vi "tester1.vi"() -> ()   [LabVIEW 2009]
panel:
  out "Column Headers":T1
  out "2D Data Array":string[][](array[string])
  in  "Run Name":string
  in  "Valve Name":string
  in  "Board Name":string
  in  "Waveform Array Input":T2(array[cluster])
  out "Waveform Array":T3(array[cluster])
  in  "Build Interval (ms)":dbl
  in  "Waveform Input":waveform(dbl)
  in  "Max Elapsed Build Time (ms)":dbl
  out "concatenated string":string
  in  "Clear Trigger SP Latch":bool=TRUE
  out "PASS/FAIL Value":bool
  in  "Clear PASS/FAIL Selection":bool
  out "FAIL Pulse":bool
  out "PASS Pulse":bool
  out "PASS OR FAIL Pulse":bool
  in  "FAIL Button":bool
  in  "PASS Button":bool
  out "Waveform Output":waveform(dbl)
  in  "High Trigger SP (VDC)":dbl
  out "Elapsed ms":dbl
  in  "y":i32
  out "Loops/Second":dbl
  out "Loop Count":i32
  out "Y":dbl[](array[numeric])
  out "Waveform Chart 2":waveform(dbl)(graph)
  in  "E-STOP Input":bool
  in  "Module Configure":T4={"DAQ #"=1, "Module #"=4, "Samples"=1000, "Mode"=10178, "Rate (Hz)"=1000.0, "Min VDC"=-10.0, "Max VDC"=32.0, "Module Type"=enum."CDAQ"} {"Rate (Hz)" format="%0.2f"; "Mode" items=["Finite Samples"=10178, "Continuous Samples"=10123, "Hardware Timed Single Point"=12522]}
  out "Task OUT":refnum<k21>="cDAQ1Mod4"
  out "Error OUT":errorcluster
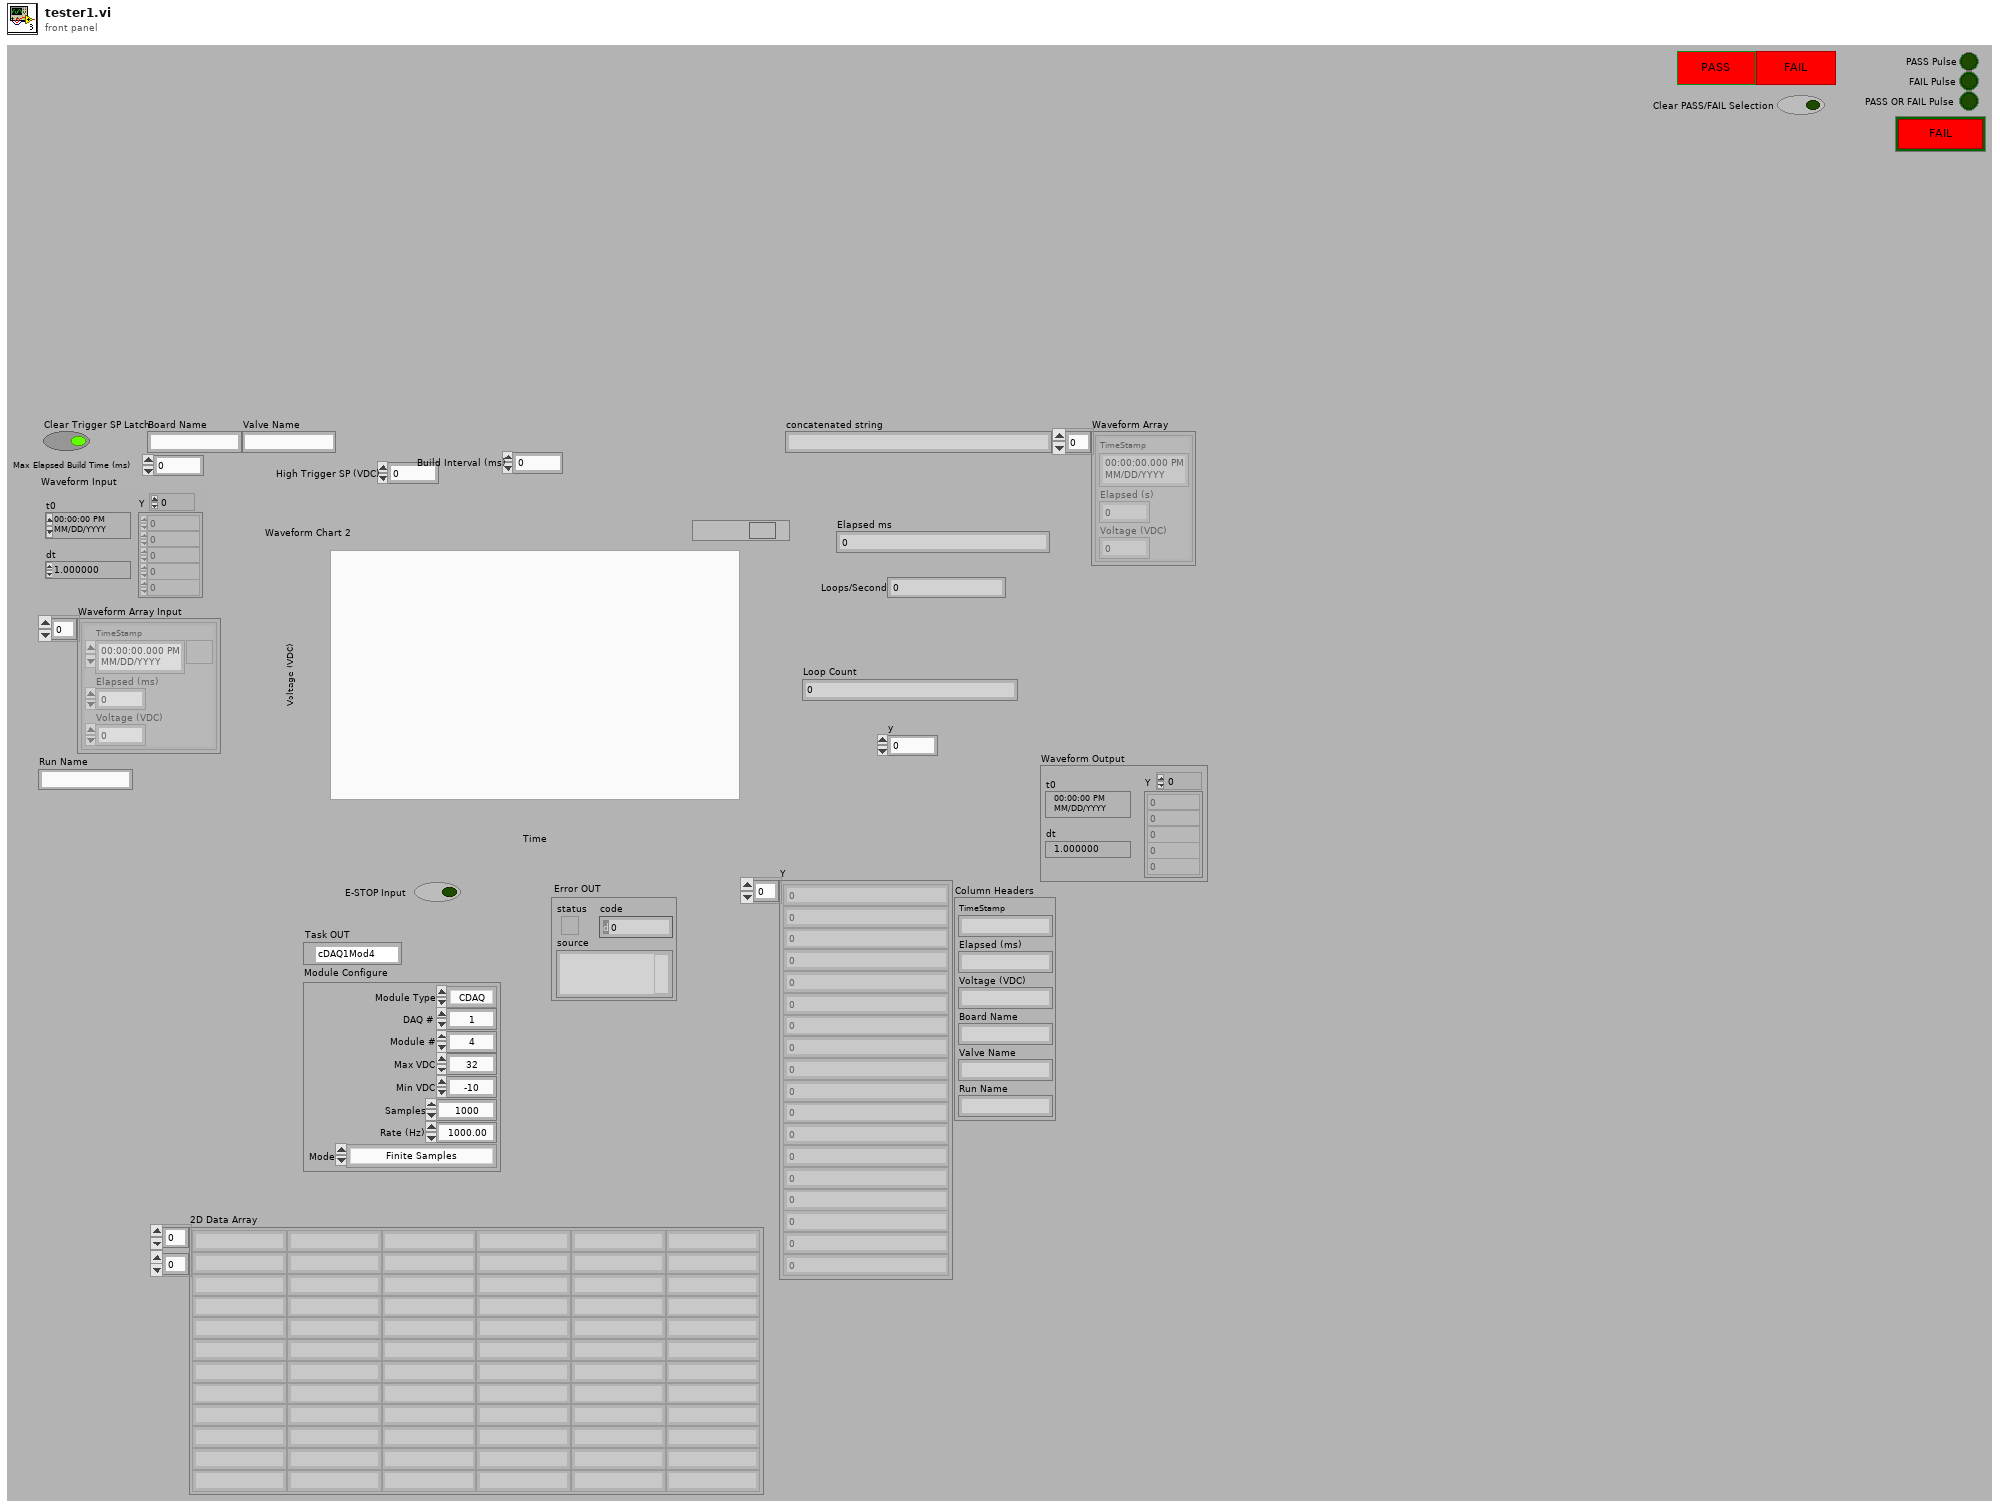
[diagram p1: front panel]
types:
  T1 = cluster{"TimeStamp":string, "Elapsed (ms)":string, "Voltage (VDC)":string, "Board Name":string, "Valve Name":string, "Run Name":string}
  T2 = cluster{"TimeStamp":timestamp, "Elapsed (ms)":dbl, "Voltage (VDC)":dbl}[]
  T3 = cluster{"TimeStamp":timestamp, "Elapsed (s)":dbl, "Voltage (VDC)":dbl}[]
  T4 = cluster{"DAQ #":i32, "Module #":i32, "Samples":i32, "Mode":i32, "Rate (Hz)":dbl, "Min VDC":dbl, "Max VDC":dbl, "Module Type":enum16{"CDAQ", "SCXI"}}
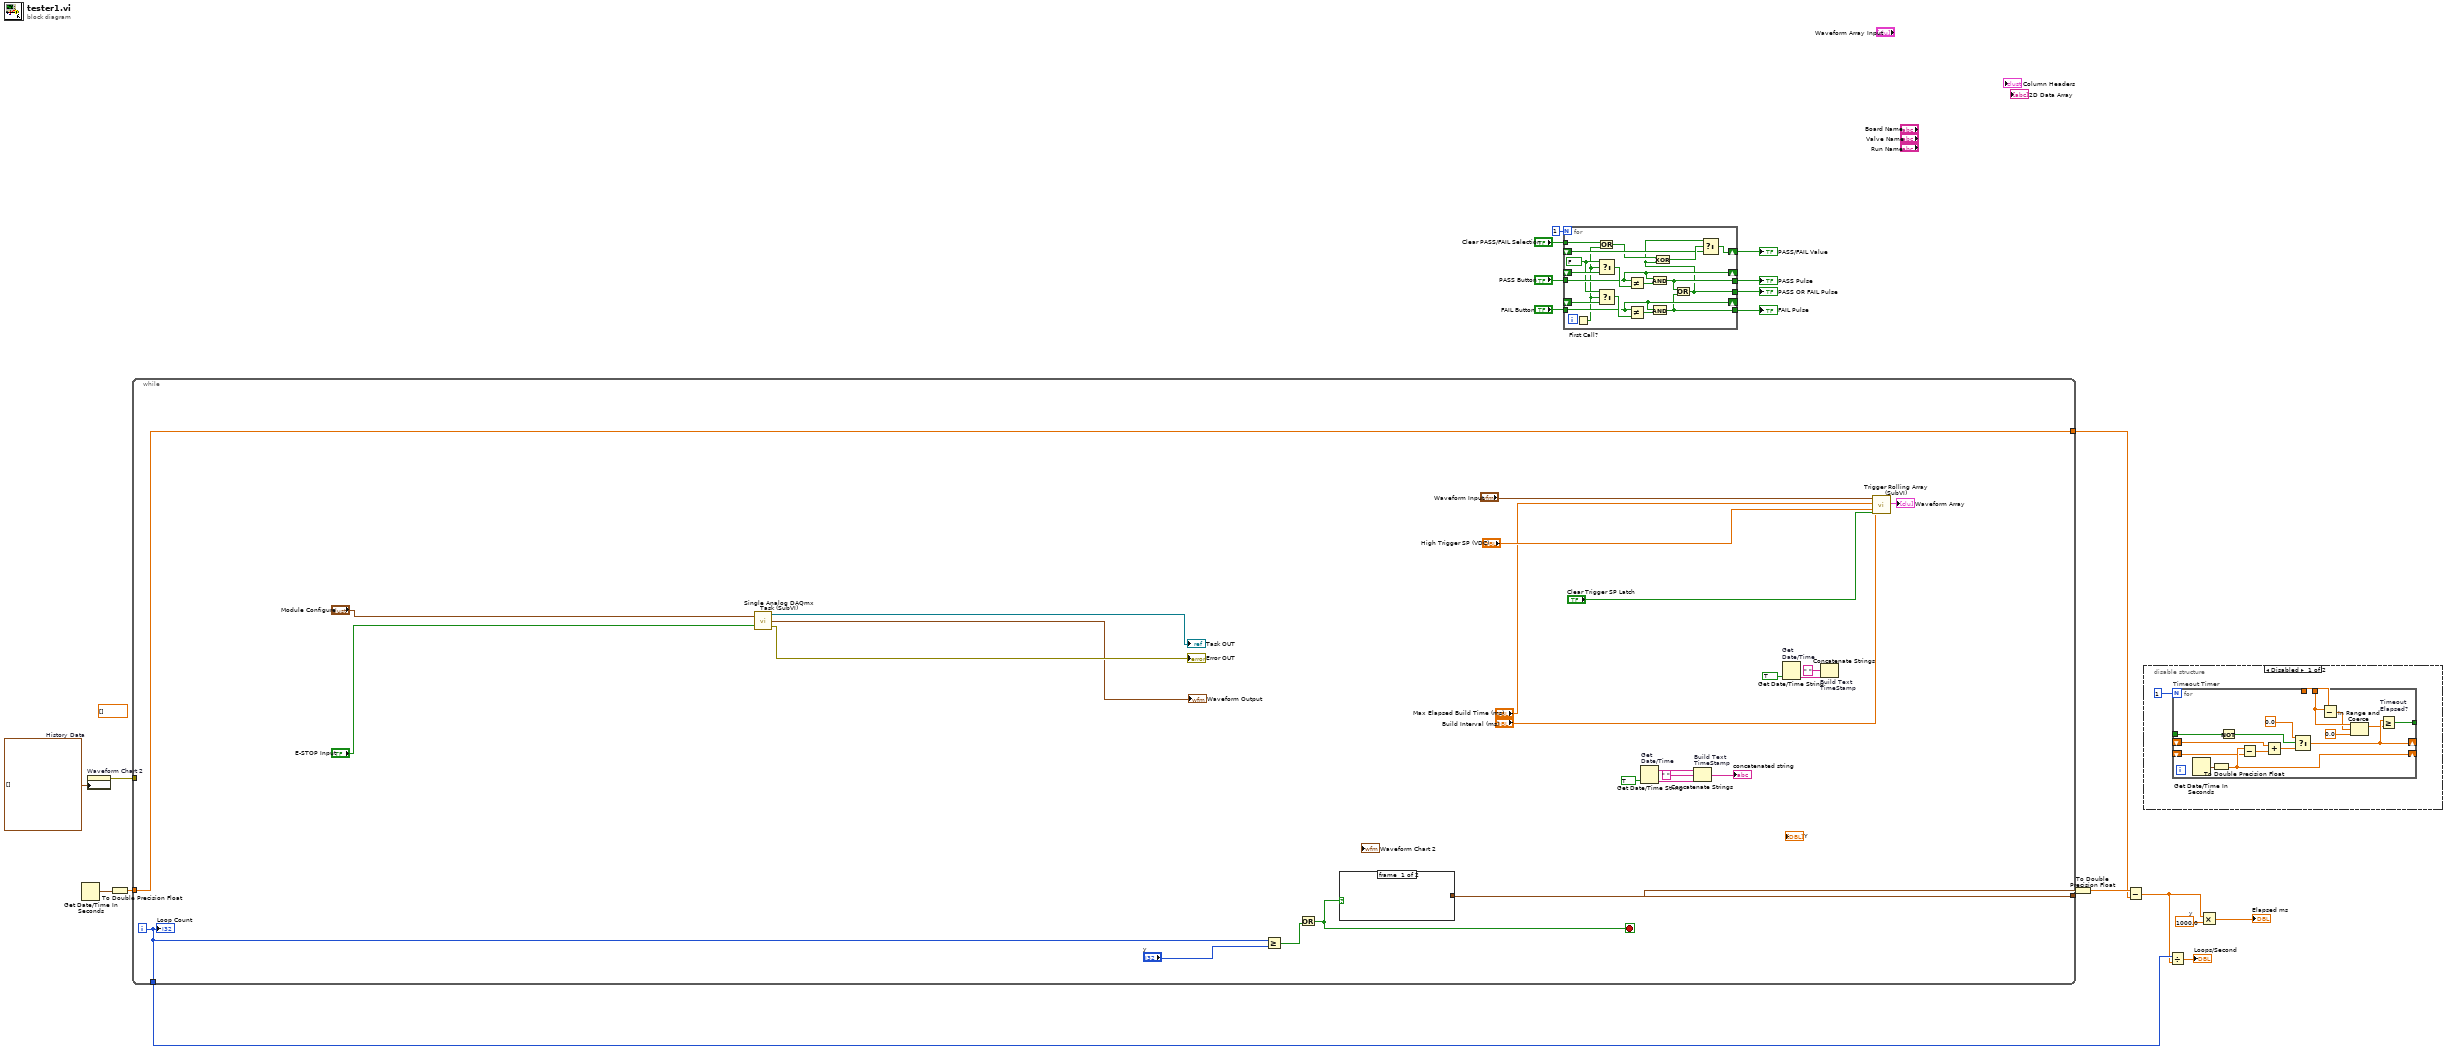
[diagram p0: block diagram]
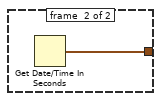
[diagram p3: hidden frame]
diagram:
  w10 = 1000.0  # y
  w19 = waveform(dbl)[] []  # History Data
  (unwired) dbl[] []
  n1 = Get Date/Time In Seconds() -> (seconds since 1Jan1904=w18:timestamp)
  n2 = property on="Waveform Chart 2" class="WFChart (strict)"("History Data"=w19) -> (error out=w20:errorcluster)  [unwired: 2 in, 1 out]
  n3 = To Double Precision Float(number=w18) -> (double precision float=w17:dbl)
  n4 = while {
    tunnel: w20 -> [_]
    tunnel: w17 -> [w44]
    tunnel: [w44] -> w14
    tunnel: [w43] -> w16
    tunnel: [w39] -> w12
    i -> [w39]
    stop <- w38 stop-if-true
    n5 = call "Single Analog DAQmx Task (SubVI).vi"("Module Configure"="Module Configure", "E-STOP Input"="E-STOP Input") -> ("Task OUT"=→"Task OUT":refnum<k21>, "Waveform Output"=→"Waveform Output":waveform(dbl), "Error OUT"=→"Error OUT":errorcluster)
    n6 = Greater Or Equal?(x=w39, y="y") -> (x >= y?=w41:bool)
    n7 = Or(y=w41) -> (x .or. y?=w38:bool)  [unwired: 1 in]
    n8 = case shown="True" w38 {
      tunnel: [_ w46] -> w43
      frame #0 {
      }
      frame #1 {
        n9 = Get Date/Time In Seconds() -> (seconds since 1Jan1904=w46:timestamp)
      }
    }
    n10 = Get Date/Time String "Get \nDate/Time"(want seconds? (F)=TRUE) -> (date string=w32:string, time string=w35:string)  [unwired: 2 out]
    n11 = Concatenate Strings "Build Text\nTimeStamp"(w32, " " ("string"), w35) -> (→"concatenated string":string)
    n12 = Get Date/Time String "Get \nDate/Time"(want seconds? (F)=TRUE) -> (time string=w26:string)  [unwired: 3 out]
    n13 = Concatenate Strings "Build Text\nTimeStamp"(" " ("string"), w26) -> ()  [unwired: 1 in, 1 out]
    n14 = call "Trigger Rolling Array (SubVI).vi"("Waveform Input"="Waveform Input", "Build Interval (ms)"="Build Interval (ms)", "Max Elapsed Build Time (ms)"="Max Elapsed Build Time (ms)", "High Trigger SP (VDC)"="High Trigger SP (VDC)", "Clear Trigger SP Latch"="Clear Trigger SP Latch") -> ("Waveform Array"=→"Waveform Array":T2)  [unwired: 14 in]
    "Loop Count" <- w39
  }
  n15 = for {
    N: 1 -> [_]
    tunnel: "PASS Button" -> [w61]
    tunnel: "FAIL Button" -> [w57]
    shift-right: [w61] -> _
    shift-left: _ -> [w64]
    tunnel: [w55] -> w6
    tunnel: [w54] -> w7
    shift-right: [w57] -> _
    shift-left: _ -> [w58]
    tunnel: [w47] -> w5
    shift-right: [w52] -> w1
    shift-left: _ -> [w51]
    tunnel: "Clear PASS/FAIL Selection" -> [w49]
    w56 = FALSE ("t")
    n16 = First Call?() -> (First Call?: T/F=w50:bool)
    n17 = Or(x=w49, y=w50) -> (x .or. y?=w48:bool)
    n18 = Select(t=w56, s=w50, f=w64) -> (s? t:f=w63:bool)
    n19 = Select(t=w56, s=w50, f=w58) -> (s? t:f=w60:bool)
    n20 = Not Equal?(x=w61, y=w63) -> (x != y?=w62:bool)
    n21 = Not Equal?(x=w57, y=w60) -> (x != y?=w59:bool)
    n22 = And(x=w61, y=w62) -> (x .and. y?=w55:bool)
    n23 = And(x=w57, y=w59) -> (x .and. y?=w54:bool)
    n24 = Or(x=w55, y=w54) -> (x .or. y?=w47:bool)
    n25 = Exclusive Or(1:w47, 2:w48) -> (0:w53:bool)
    n26 = Select(t=w47, s=w53, f=w51) -> (s? t:f=w52:bool)
  }
  "PASS OR FAIL Pulse" <- w5
  "PASS Pulse" <- w6
  "FAIL Pulse" <- w7
  "PASS/FAIL Value" <- w1
  n27 = To Double Precision Float(number=w16) -> (double precision float=w15:dbl)
  n28 = Subtract(x=w15, y=w14) -> (x-y=w11:dbl)
  n29 = disable-structure shown="Disabled" {
    frame #0 {
      n30 = for "Timeout Timer" {
        N: 1 -> [_]
        shift-right: [w71] -> _
        shift-left: _ -> [w81]
        shift-right: [w79] -> _
        shift-left: _ -> [w78]
        tunnel: [w73] -> _
        tunnel: _ -> [w76]
        tunnel: _ -> [w69]
        tunnel: _ -> [w70]
        n31 = Get Date/Time In Seconds() -> (seconds since 1Jan1904=w80:timestamp)
        n32 = To Double Precision Float(number=w80) -> (double precision float=w79:dbl)
        n33 = Not(x=w76) -> (.not. x?=w75:bool)
        n34 = Subtract(x=w79, y=w78) -> (x-y=w77:dbl)
        n35 = Add(x=w81, y=w77) -> (x+y=w74:dbl)
        n36 = Select(t=0.0, s=w75, f=w74) -> (s? t:f=w71:dbl)
        n37 = Subtract(x=w69, y=w70) -> (x-y=w67:dbl)
        n38 = In Range and Coerce(upper limit=w69, x=w67, lower limit=0.0) -> (coerced(x)=w66:dbl)  [unwired: 1 out]
        n39 = Greater Or Equal? "Timeout\nElapsed?"(x=w71, y=w66) -> (x >= y?=w73:bool)
      }
    }
    frame #1 {
    }
  }
  n40 = Divide(x=w12, y=w11) -> (x/y=→"Loops/Second":dbl)
  n41 = Multiply(x=w11, y=w10) -> (x*y=→"Elapsed ms":dbl)
